vi "test Acyclic Loopback Multiple Pretrigger Writes.vi"(8 "error in":errorcluster, 11 "TestCase in":refnum<class "Single Board 1Ch Loopback.lvclass">) -> (0 "error out":errorcluster, 3 "TestCase out":refnum<class "Single Board 1Ch Loopback.lvclass">)   [LabVIEW 2020, in "Single Board 1Ch Loopback.lvclass"]
uses:
  Single Board 1Ch Loopback.lvclass
  C:/dev/git/niveristand-custom-device-testing-tools/VeriStandTestCase/VeriStandTestCase.lvclass
  <vilib>/numeric/Random Number (Range) U64.vi
  <vilib>/numeric/sub_Random U32.vi
  <vilib>/NI VeriStand/Execution/Workspace/NI VeriStand - Set Multiple Channel Values.vi
  <vilib>/addons/_JKI Toolkits/VI Tester/TestCase.llb/TestCase.lvclass
  <vilib>/NI VeriStand/Execution/Workspace/NI_VS Workspace ExecutionAPI.lvlib
  niveristand-custom-device-testing-tools/VeriStandTestUtilities/VeriStandTestUtilities.lvlib
  C:/Program Files (x86)/National Instruments/LabVIEW 2020/vi.lib/addons/_JKI Toolkits/VI Tester/TestCase.llb/TestCase.lvclass
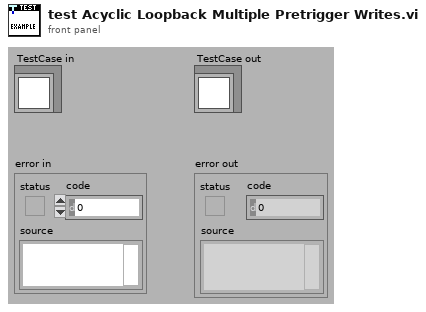
[diagram p1: front panel]
types:
  T1 = typedef "NI_VS Workspace ExecutionAPI.lvlib/WorkspaceAPI.ctl" = refnum<k24>
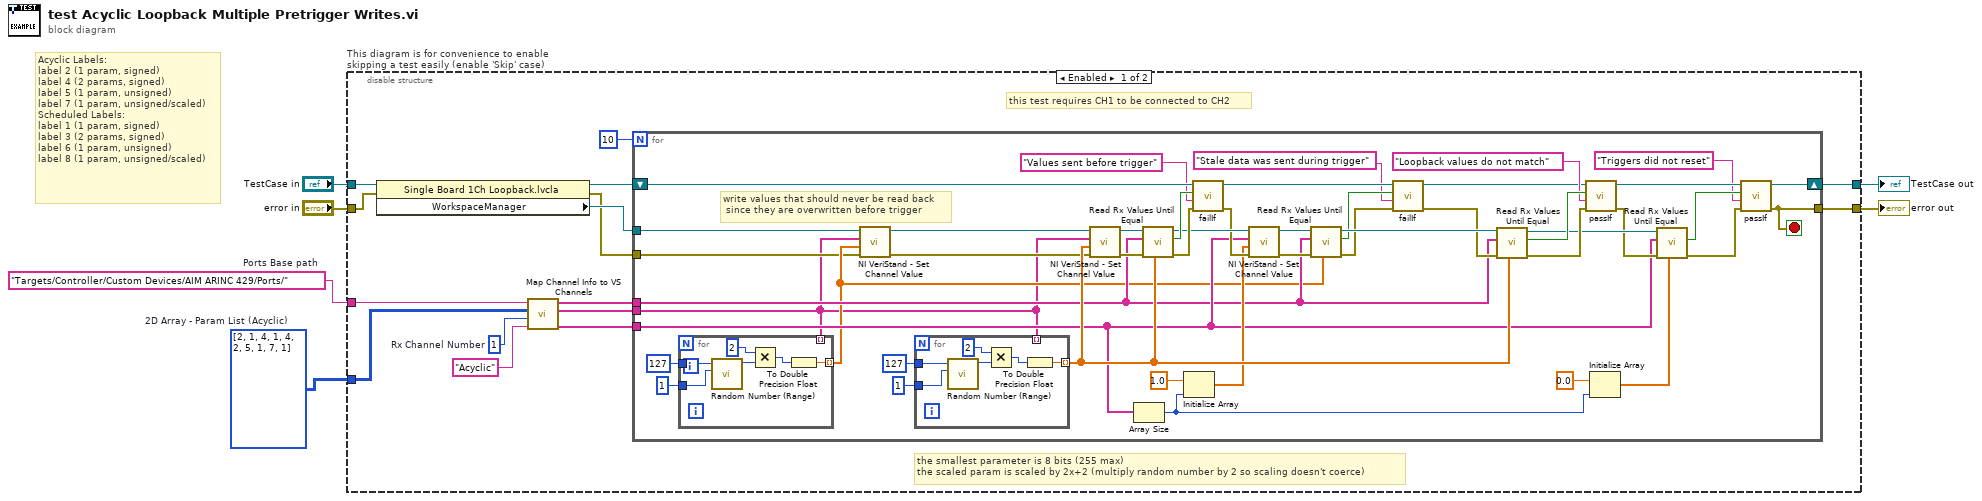
[diagram p0: block diagram]
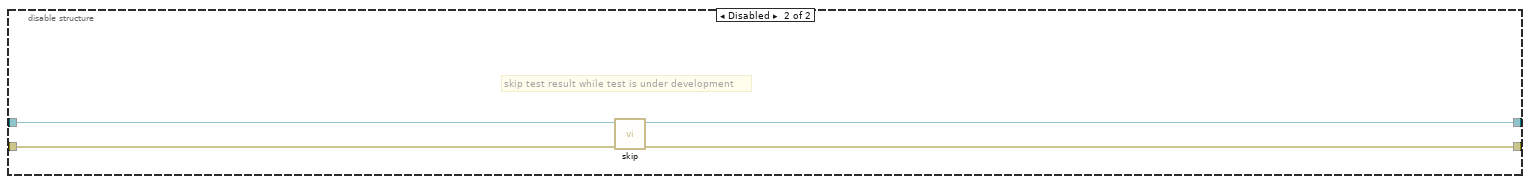
[diagram p2: hidden frame]
diagram:
  w2 = i32[][] [[2, 1], [4, 1], [4, 2], [5, 1], [7, 1]]  # 2D Array - Param List (Acyclic)
  w3 = "Targets/Controller/Custom Devices/AIM ARINC 429/Ports/"  # Ports Base path
  # "Acyclic Labels:\nlabel 2 (1 param, signed)\nlabel 4 (2 params, signed)\nlabel 5 (1 param, unsigned)\nlabel 7 (1 param, unsigned/scaled)\nScheduled Labels:\nlabel 1 (1 param, signed)\nlabel 3 (2 params, signed)\nlabel 6 (1 param, unsigned)\nlabel 8 (1 param, unsigned/scaled)"
  n1 = disable-structure "This diagram is for convenience to enable skipping a test easily (enable 'Skip' case)" shown="Enabled" {
    disable-tunnel: "TestCase in" -> [w15 w83]
    disable-tunnel: [w13 w81] -> w1
    disable-tunnel: [w12 w82] -> w5
    disable-tunnel: "error in" -> [w14 w80]
    disable-tunnel: w3 -> [w16 _]
    disable-tunnel: w2 -> [w9 _]
    frame Enabled {
      w10 = 1  # Rx Channel Number
      # "this test requires CH1 to be connected to CH2"
      # "the smallest parameter is 8 bits (255 max)\nthe scaled param is scaled by 2x+2 (multiply random number by 2 so scaling doesn't coerce)"
      n2 = property class="Single Board 1Ch Loopback.lvcla"(reference=w15, error in=w14) -> (reference out=w18:refnum<class "Single Board 1Ch Loopback.lvclass">, error out=w19:errorcluster, "WorkspaceManager"=w20:T1)
      n3 = call "Map Channel Info to VS Channels.vi"("Transfer Type"="Acyclic", "Rx Channel Number"=w10, "2D Array - Label/Param List"=w9, "VS Channel Base Port"=w16) -> ("Tx Trigger Channels Array"=w7:string[], "Tx Channels Array"=w8:string[], "Rx Channels Array"=w21:string[])  [unwired: 4 in, 1 out]
      n4 = for {
        N: 10 -> [_]
        tunnel: w21 -> [w29]
        tunnel: w20 -> [w26]
        tunnel: w19 -> [w23]
        tunnel: w8 -> [w22]
        shift-right: [w53] -> w13
        shift-left: w18 -> [w62]
        tunnel: [w55] -> w12
        tunnel: w7 -> [w43]
        stop <- w55 stop-if-true
        # "write values that should never be read back\n since they are overwritten before trigger"
        n5 = for {
          tunnel: [w72] -> w28 mode=indexing
          tunnel: u64 127 ("upper bound (100)") -> [w71]
          tunnel: u64 1 ("upper bound (100)") -> [w70]
          tunnel: w22 -> [_] mode=indexing
          n6 = call-poly <vilib>:"Random Number (Range).vi"("lower bound (0)"=w70, "upper bound (100)"=w71) -> ("number"=w73:u64)  [unwired: 9 in]
          n7 = Multiply(x=u64 2, y=w73) -> (x*y=w69:u64)
          n8 = To Double Precision Float(number=w69) -> (double precision float=w72:dbl)
        }
        n9 = call-poly <vilib>:"NI VeriStand - Set Channel Value.vi"("error in (no error)"=w23, "Values"=w28, "Channels"=w22, "WorkspaceManager in"=w26) -> ("error out"=w24:errorcluster, "WorkspaceManager out"=w25:T1)  [unwired: 6 in]
        n10 = for {
          tunnel: [w78] -> w58 mode=indexing
          tunnel: u64 127 ("upper bound (100)") -> [w77]
          tunnel: u64 1 ("upper bound (100)") -> [w76]
          tunnel: w22 -> [_] mode=indexing
          n11 = call-poly <vilib>:"Random Number (Range).vi"("lower bound (0)"=w76, "upper bound (100)"=w77) -> ("number"=w79:u64)  [unwired: 9 in]
          n12 = Multiply(x=u64 2, y=w79) -> (x*y=w75:u64)
          n13 = To Double Precision Float(number=w75) -> (double precision float=w78:dbl)
        }
        n14 = call-poly <vilib>:"NI VeriStand - Set Channel Value.vi"("error in (no error)"=w24, "Values"=w58, "Channels"=w22, "WorkspaceManager in"=w25) -> ("error out"=w63:errorcluster, "WorkspaceManager out"=w65:T1)  [unwired: 6 in]
        n15 = Array Size(array=w43) -> (size(s)=w40:i32)
        n16 = call "Read Rx Values Until Equal.vi"("expected values"=w58, "error in"=w63, "Rx aliases"=w29, "workspace manager in"=w65) -> ("error out"=w64:errorcluster, "values equal expected"=w61:bool, "workspace manager out"=w60:T1)  [unwired: 5 in]
        n17 = Initialize Array(1.0, w40) -> (w44:dbl[])
        n18 = call-dynamic "failIf.vi"("error in (no error)"=w64, "message (\"\")"="Values sent before trigger" ("message (\"\")"), "fail"=w61, "TestCase in"=w62) -> ("error out"=w59:errorcluster, "TestCase out"=w34:refnum<class "Single Board 1Ch Loopback.lvclass">)  [unwired: 6 in]
        n19 = call-poly <vilib>:"NI VeriStand - Set Channel Value.vi"("error in (no error)"=w59, "Values"=w44, "Channels"=w43, "WorkspaceManager in"=w60) -> ("error out"=w37:errorcluster, "WorkspaceManager out"=w36:T1)  [unwired: 6 in]
        n20 = call "Read Rx Values Until Equal.vi"("expected values"=w28, "error in"=w37, "Rx aliases"=w29, "workspace manager in"=w36) -> ("error out"=w32:errorcluster, "values equal expected"=w30:bool, "workspace manager out"=w35:T1)  [unwired: 5 in]
        n21 = call-dynamic "failIf.vi"("error in (no error)"=w32, "message (\"\")"="Stale data was sent during trigger" ("message (\"\")"), "fail"=w30, "TestCase in"=w34) -> ("error out"=w31:errorcluster, "TestCase out"=w33:refnum<class "Single Board 1Ch Loopback.lvclass">)  [unwired: 6 in]
        n22 = call "Read Rx Values Until Equal.vi"("expected values"=w58, "error in"=w31, "Rx aliases"=w29, "workspace manager in"=w35) -> ("error out"=w56:errorcluster, "values equal expected"=w57:bool, "workspace manager out"=w51:T1)  [unwired: 5 in]
        n23 = call-dynamic "passIf.vi"("error in (no error)"=w56, "message (\"\")"="Loopback values do not match" ("message (\"\")"), "pass"=w57, "TestCase in"=w33) -> ("error out"=w50:errorcluster, "TestCase out"=w54:refnum<class "Single Board 1Ch Loopback.lvclass">)  [unwired: 6 in]
        n24 = Initialize Array(0.0, w40) -> (w41:dbl[])
        n25 = call "Read Rx Values Until Equal.vi"("expected values"=w41, "error in"=w50, "Rx aliases"=w43, "workspace manager in"=w51) -> ("error out"=w49:errorcluster, "values equal expected"=w52:bool)  [unwired: 5 in, 1 out]
        n26 = call-dynamic "passIf.vi"("error in (no error)"=w49, "message (\"\")"="Triggers did not reset" ("message (\"\")"), "pass"=w52, "TestCase in"=w54) -> ("error out"=w55:errorcluster, "TestCase out"=w53:refnum<class "Single Board 1Ch Loopback.lvclass">)  [unwired: 6 in]
      }
    }
    frame Disabled {
      # "skip test result while test is under development"
      n27 = call <vilib>:"skip.vi"("error in (no error)"=w80, "TestCase in"=w83) -> ("error out"=w82:errorcluster, "TestCase out"=w81:refnum<class "Single Board 1Ch Loopback.lvclass">)  [unwired: 8 in]
    }
  }
  "error out" <- w5
  "TestCase out" <- w1
